vi "WLAN Fetch TxP.vi"(0 "Instrument Handle In":refnum<k21>, 1 "Selector String":string, 11 "error in (no error)":errorcluster) -> (4 "Instrument Handle Out":refnum<k21>, 6 "TxP Results":T1 {"Average Power Mean (dBm)" format="%.2f"; "Peak Power Maximum (dBm)" format="%.2f"}, 15 "error out":errorcluster)   [LabVIEW 2016, in "RFmxWLAN.lvlib"]
uses:
  RFmxWLAN.lvlib
  Typedefs/WLAN TxP Results.ctl
  <vilib>/RFmx/WLAN/mx/RFmxWLAN.llb/RFmxWLAN TXP Fetch Power Trace.vi
  <vilib>/RFmx/WLAN/mx/RFmxWLAN.llb/RFmxWLAN TXP Fetch Measurement.vi
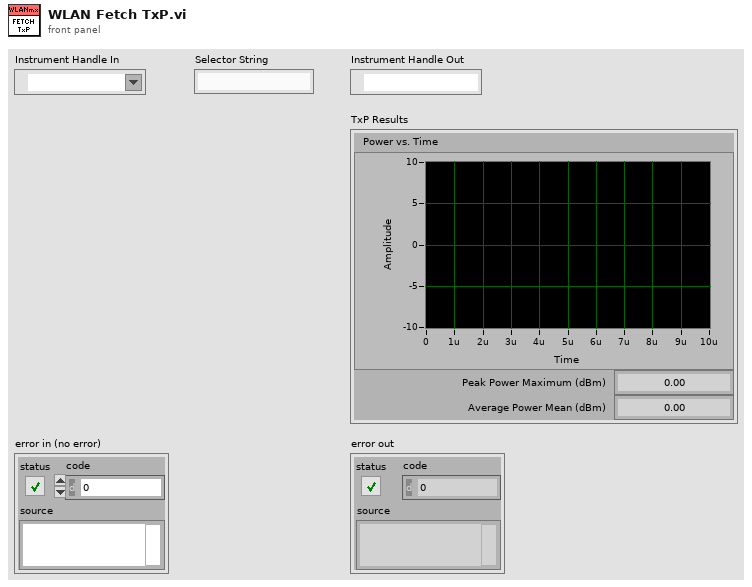
[diagram p1: front panel]
types:
  T1 = typedef "RFmxWLAN.lvlib/WLAN TxP Results.ctl" = cluster{"Power vs. Time":cluster{"x0":dbl, "dx":dbl, "y":sgl[]}, "Peak Power Maximum (dBm)":dbl, "Average Power Mean (dBm)":dbl}
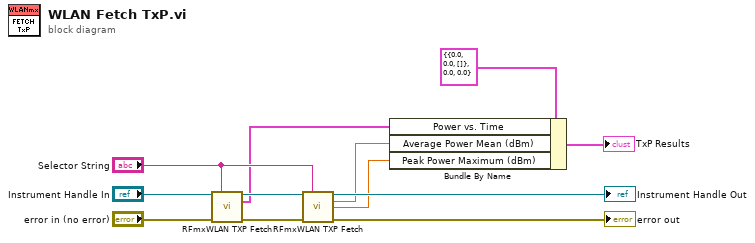
[diagram p0: block diagram]
diagram:
  n1 = call-poly <vilib>:"RFmxWLAN TXP Fetch.vi"("Instrument Handle In"="Instrument Handle In", "Selector String"="Selector String", "error in (no error)"="error in (no error)") -> ("Instrument Handle Out"=w8:refnum<k21>, "Power (dBm)"=w3:cluster{"x0":dbl, "dx":dbl, "y":sgl[]}, "error out"=w11:errorcluster)  [unwired: 10 in]
  n2 = call-poly <vilib>:"RFmxWLAN TXP Fetch.vi"("Instrument Handle In"=w8, "Selector String"="Selector String", "error in (no error)"=w11) -> ("Instrument Handle Out"=→"Instrument Handle Out":refnum<k21>, "Average Power Mean (dBm)"=w2:dbl, "Peak Power Maximum (dBm)"=w1:dbl, "error out"=→"error out":errorcluster)  [unwired: 9 in]
  n3 = Bundle By Name(cluster=T1 {"Power vs. Time"={"x0"=0.0, "dx"=0.0, "y"=[]}, "Peak Power Maximum (dBm)"=0.0, "Average Power Mean (dBm)"=0.0} ("WLAN TxP Results"), "Power vs. Time"=w3, "Average Power Mean (dBm)"=w2, "Peak Power Maximum (dBm)"=w1) -> (→"TxP Results":T1)
